vi "pointToSegmnetDist.vi"(10 "point":cluster{"X":sgl, "Y":sgl}, 11 "Line Segment":T1) -> (0 "t":dbl, 1 "onSegment":bool, 3 "distance":dbl, 4 "y-dist":dbl, 6 "x-Dist":dbl)   [LabVIEW 2015]
uses:
  <vilib>/Analysis/baseanly.llb/Real Dot Product.vi
  <vilib>/Analysis/NI_AALBase.lvlib
panel:
  out "lineDistance":sgl
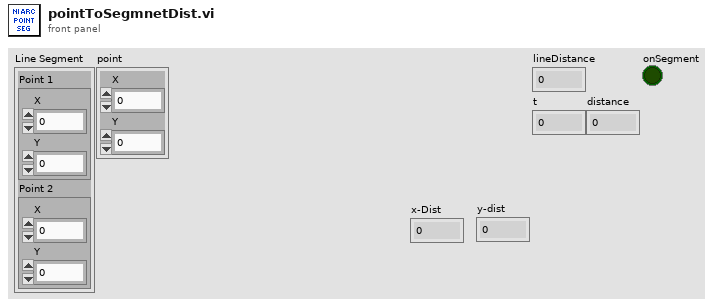
[diagram p1: front panel]
types:
  T1 = cluster{"Point 1":cluster{"X":sgl, "Y":sgl}, "Point 2":cluster{"X":sgl, "Y":sgl}}
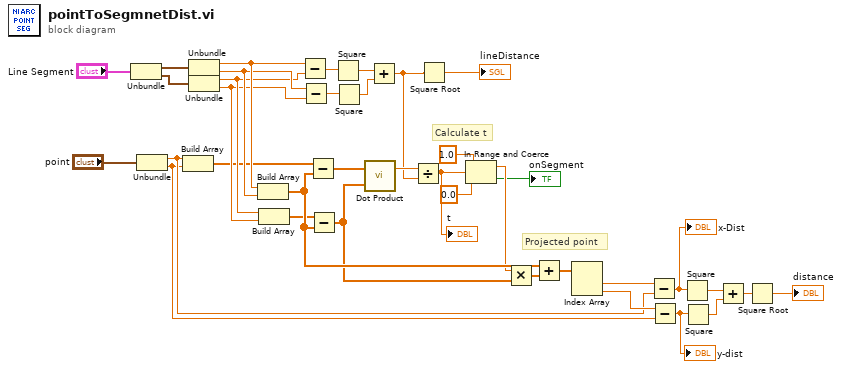
[diagram p0: block diagram]
diagram:
  # "Projected point"
  # "Calculate t"
  n1 = Unbundle("Line Segment") -> ("Point 1"=w36:cluster{"X":sgl, "Y":sgl}, "Point 2"=w35:cluster{"X":sgl, "Y":sgl})
  n2 = Unbundle("point") -> ("X"=w9:sgl, "Y"=w8:sgl)
  n3 = Build Array(w9, w8) -> (w25:sgl[])
  n4 = Unbundle(w36) -> ("X"=w29:sgl, "Y"=w28:sgl)
  n5 = Unbundle(w35) -> ("X"=w27:sgl, "Y"=w26:sgl)
  n6 = Build Array(w29, w28) -> (w20:sgl[])
  n7 = Build Array(w27, w26) -> (w18:sgl[])
  n8 = Subtract(x=w29, y=w27) -> (x-y=w34:sgl)
  n9 = Subtract(x=w28, y=w26) -> (x-y=w33:sgl)
  n10 = Subtract(x=w25, y=w20) -> (x-y=w24:sgl[])
  n11 = Subtract(x=w18, y=w20) -> (x-y=w16:sgl[])
  n12 = Square(x=w34) -> (x^2=w32:sgl)
  n13 = Square(x=w33) -> (x^2=w31:sgl)
  n14 = call-poly <vilib>:"Dot Product.vi"("Y Vector"=w16, "X Vector"=w24) -> ("X * Y"=w23:dbl)  [unwired: 1 out]
  n15 = Add(x=w32, y=w31) -> (x+y=w2:sgl)
  n16 = Divide(x=w23, y=w2) -> (x/y=w5:dbl)
  "t" <- w5
  n17 = Square Root(x=w2) -> (sqrt(x)=→"lineDistance":sgl)
  n18 = In Range and Coerce(upper limit=1.0, x=w5, lower limit=0.0) -> (coerced(x)=w19:dbl, In Range?=→"onSegment":bool)
  n19 = Multiply(x=w19, y=w16) -> (x*y=w17:dbl[])
  n20 = Add(x=w20, y=w17) -> (x+y=w15:dbl[])
  n21 = Index Array(array=w15) -> (element #1=w11:dbl, element #2=w10:dbl)  [unwired: 2 in]
  n22 = Subtract(x=w11, y=w9) -> (x-y=w12:dbl)
  "x-Dist" <- w12
  n23 = Subtract(x=w10, y=w8) -> (x-y=w3:dbl)
  "y-dist" <- w3
  n24 = Square(x=w12) -> (x^2=w13:dbl)
  n25 = Square(x=w3) -> (x^2=w14:dbl)
  n26 = Add(x=w13, y=w14) -> (x+y=w7:dbl)
  n27 = Square Root(x=w7) -> (sqrt(x)=→"distance":dbl)
